vi "simple_graph.vi"() -> ()   [LabVIEW 2013]
panel:
  in  "opóŸnienie":dbl
  out "Waveform Chart":cluster{dbl, dbl}(graph)
  out "wartoœæ srednia 3 losowych":dbl
  in  "stop":bool
  in  "zakres do":dbl
  in  "zakres od":dbl
  out "losowa":dbl
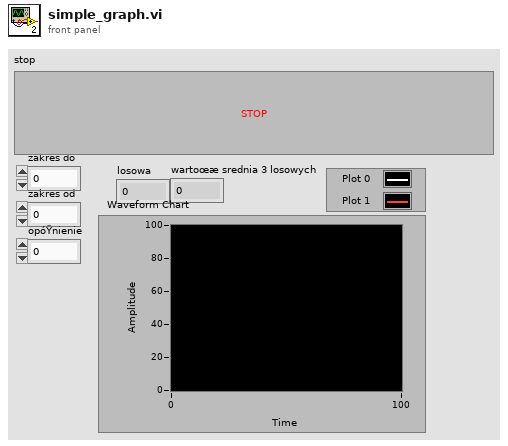
[diagram p1: front panel]
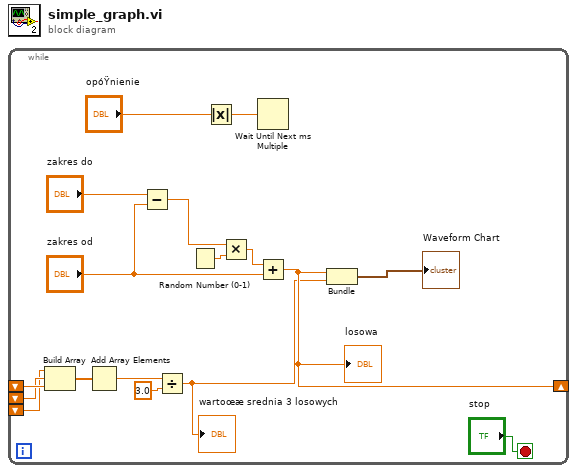
[diagram p0: block diagram]
diagram:
  n1 = while {
    shift-right: [w4] -> _
    shift-left: _ -> [w11]
    shift-left: _ -> [w10]
    shift-left: _ -> [w9]
    stop <- "stop" stop-if-true
    n2 = Build Array(w9, w10, w11) -> (w8:dbl[])
    n3 = Add Array Elements(numeric array=w8) -> (sum=w7:dbl)
    n4 = Subtract(x="zakres do", y="zakres od") -> (x-y=w15:dbl)
    n5 = Divide(x=w7, y=3.0) -> (x/y=w3:dbl)
    "wartoœæ srednia 3 losowych" <- w3
    n6 = Random Number (0-1)() -> (number: 0 to 1=w16:dbl)
    n7 = Absolute Value(x="opóŸnienie") -> (abs(x)=w1:dbl)
    n8 = Multiply(x=w15, y=w16) -> (x*y=w17:dbl)
    n9 = Wait Until Next ms Multiple(millisecond multiple=w1) -> ()  [unwired: 1 out]
    n10 = Add(x=w17, y="zakres od") -> (x+y=w4:dbl)
    "losowa" <- w4
    n11 = Bundle(w4, w3) -> (→"Waveform Chart":cluster{dbl, dbl})  [unwired: 1 in]
  }
